vi "Sim Camera.vi"() -> ()   [LabVIEW 2012]
uses:
  Program Files (x86)/National Instruments/LabVIEW 2012/examples/robotics/Simulator/Traffic/Auto Driving/Auto Starter Kit.ctl
  <vilib>/vision/Image Controls.llb/IMAQ Image.ctl
  <vilib>/robotics/Steering/Differential Steering Frame/NI_Robotics_Differential Steering Frame.lvclass
  <instrlib>/DC Motor Controller/HAIOL/DC Motor Controller.lvclass
  <vilib>/Platform/TimedLoop/XDataNode/timing_clust.ctl
  <vilib>/Platform/TimedLoop/XDataNode/nitl_modes.ctl
  <vilib>/Platform/TimedLoop/XDataNode/wakeup.ctl
  <vilib>/robotics/Simulator/Interface/Simulator References/Get Sensor Reference.vi
  <vilib>/Platform/TimedLoop/XDataNode/XDataNode.xnode
  <vilib>/Platform/TimedLoop/XDataNode/XDNodeRunTimeDep.lvlib
  <resource>/objmgr/LVODE.rc
  <vilib>/robotics/Simulator/NI_Robotics_Simulator.lvlib
panel:
  out "VI Name":string
  out "Camera on Starter Kit 1.0":refnum<vi>(3d-picture)
  in  "error in":errorcluster
  out "error out":errorcluster
  in  "stop?":bool caption="Stop (F)"
  out "Image Out":T1(plugin-control)
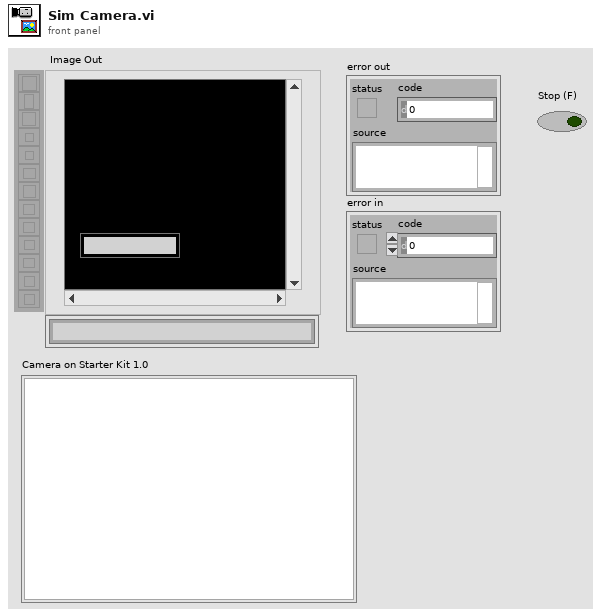
[diagram p1: front panel]
types:
  T1 = typedef "IMAQ Image.ctl" = refnum<image>
  T2 = typedef "Auto Starter Kit.ctl" = cluster{"Camera Image":T1, "Light Detect Dst":T1, "Path Detect Dst":T1, "Camera":refnum<k20>, "3D Picture":refnum<vi>, "Steering Frame":refnum<class "NI_Robotics_Differential Steering Frame.lvclass">, "Left Motor Controller":refnum<class "DC Motor Controller.lvclass">, "Right Motor Controller":refnum<class "DC Motor Controller.lvclass">}
  T3 = cluster{"Robot":string, "Sensors":string[], "Joints":string[], "Actuators":string[], "Robot Components":string[]}[]
  T4 = cluster{"Robot":string, "Sensors":string[], "Joints":string[], "Actuators":string[], "Robot Components":string[]}
  T5 = typedef "XDNodeRunTimeDep.lvlib/timing_clust.ctl" = cluster{"Expected End [f-1]":u64, "Actual End [f-1]":u64, "Finished Late? [f-1]":bool, "Expected End [i-1]":u64, "Actual End [i-1]":u64, "Finished Late? [i-1]":bool, "Expected Start [i]":u64, "Actual Start [i]":u64, "Expected Start [f]":u64, "Actual Start [f]":u64, "Source Name":string, "Structure Name":string, "Period":i64, "Deadline":i64, "Offset":i64, "Start":i64, "Priority":i32, "Timeout":i32, "Mode":T6, "Wakeup Reason":T7, "Error":errorcluster, "Source Type":string, "Secondary Source Type":string, "Global End Time":u64, "Global Start Time":u64, "Frame Duration":u64, "Iteration Duration":u64, "Assigned CPU":i32, "I/O Scan Engine Mode":u32}
  T6 = typedef "XDNodeRunTimeDep.lvlib/nitl_modes.ctl" = enum32{"No Change", "Process missed periods, maintain original phase", "Discard missed periods, maintain original phase", "Process missed periods, ignore original phase", "Discard missed periods, ignore original phase"}
  T7 = typedef "XDNodeRunTimeDep.lvlib/wakeup.ctl" = enum32{"Normal", "Aborted", "Asynchronous wakeup", "Timing source error", "Timed loop error", "Timeout"}
  T8 = cluster{"Position[0]":sgl, "Position[1]":sgl, "Position[2]":sgl}
  T9 = cluster{"Target[0]":sgl, "Target[1]":sgl, "Target[2]":sgl}
  T10 = cluster{"UpDirection[0]":sgl, "UpDirection[1]":sgl, "UpDirection[2]":sgl}
  T11 = typedef "imagedata.ctl" = cluster{"image type":i32, "image depth":i32, "image":u8[], "mask":u8[], "colors":u32[], "Rectangle":cluster{"left":i16, "top":i16, "right":i16, "bottom":i16}}
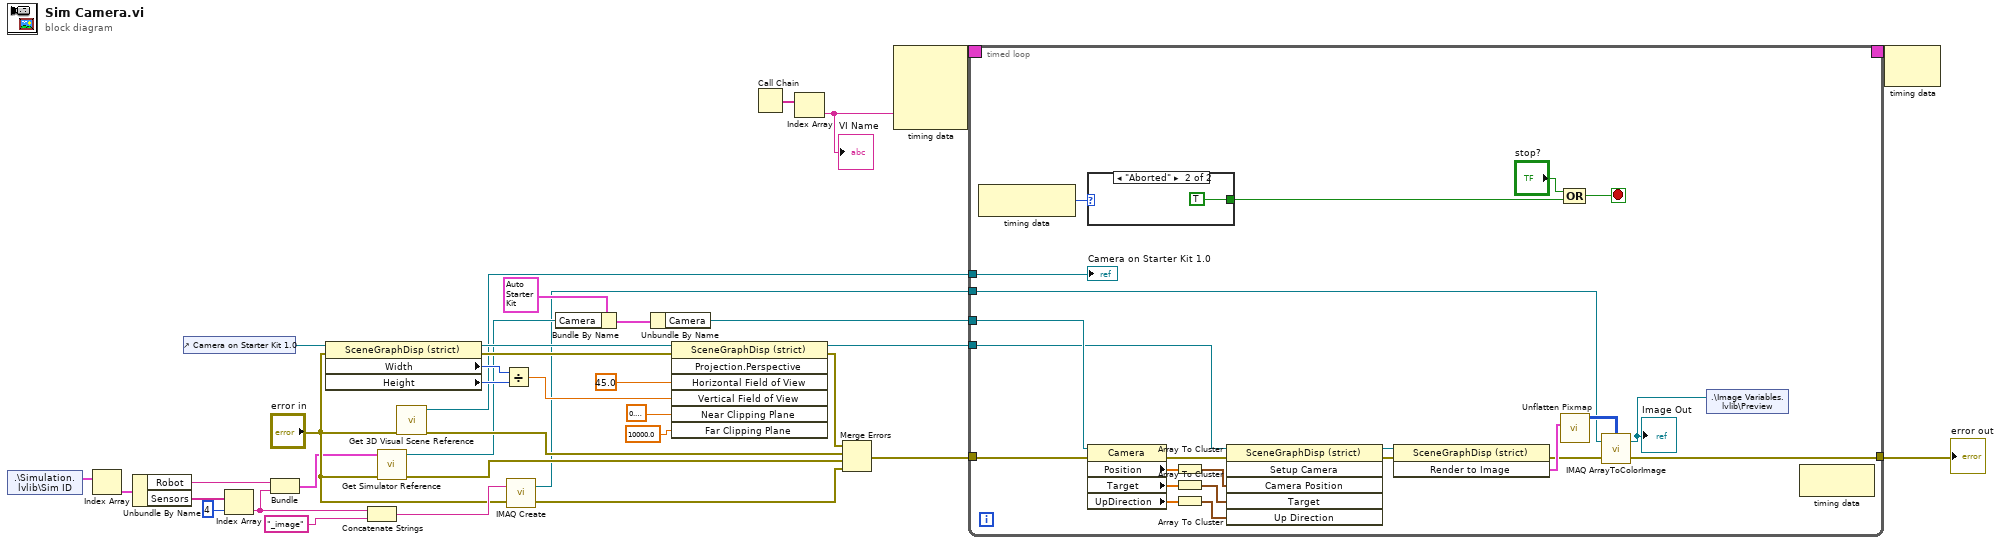
[diagram p0: block diagram]
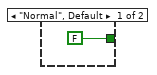
[diagram p2: hidden frame]
diagram:
  n1 = shared-variable ".\\Simulation.lvlib\\Sim ID"() -> (w9:T3)  [unwired: 1 in, 1 out]
  n2 = Index Array(array=w9) -> (element=w8:T4)  [unwired: 1 in]
  n3 = Unbundle By Name(w8) -> ("Robot"=w5:string, "Sensors"=w7:string[])
  n4 = control-ref of="Camera on Starter Kit 1.0"() -> (w25:refnum<vi>)
  n5 = Index Array(array=w7, index=4) -> (element=w4:string)
  n6 = Bundle("Robot"=w5, w4) -> (w3:cluster{"Robot":string, string})  [unwired: 1 in]
  n7 = property on="Property Node" class="SceneGraphDisp (strict)"(reference=w25, error in="error in") -> (reference out=w26:refnum<vi>, error out=w33:errorcluster, "Width"=w31:u32, "Height"=w32:u32)
  n8 = Concatenate Strings(w4, "_image" ("Image Name")) -> (w14:string)
  n9 = call-poly <vilib>:"Get Simulator Reference.vi"("error in (no error)"="error in", "device ID"=w3) -> ("error out"=w20:errorcluster, "sensor ref"=w16:refnum<k20>)  [unwired: 8 in]
  n10 = call <vilib>:"Get 3D Visual Scene Reference.vi"("error in"="error in") -> ("error out"=w22:errorcluster, "scene ref"=w24:refnum<vi>)  [unwired: 9 in]
  n11 = Divide(x=w31, y=w32) -> (x/y=w28:dbl)
  n12 = call "IMAQ Create"("Image Name"=w14, "error in (no error)"="error in") -> ("New Image"=w10:T1, "error out"=w11:errorcluster)  [unwired: 2 in, 1 out]
  n13 = Bundle By Name(cluster=T2 {"Camera Image"=refnum, "Light Detect Dst"=refnum, "Path Detect Dst"=refnum, "Camera"=refnum, "3D Picture"=refnum, "Steering Frame"=refnum, "Left Motor Controller"=refnum, "Right Motor Controller"=refnum} ("Auto Starter Kit"), "Camera"=w16) -> (w17:T2)
  n14 = Unbundle By Name(w17) -> ("Camera"=w15:refnum<k20>)
  n15 = invoke on="Invoke Node" class="SceneGraphDisp (strict)" method="Projection.Perspective"(reference=w26, error in=w33, "Horizontal Field of View"=sgl 45.0 ("Field of View"), "Vertical Field of View"=w28, "Near Clipping Plane"=sgl 0.2, "Far Clipping Plane"=sgl 10000.0) -> (reference out=w19:refnum<vi>, error out=w23:errorcluster)  [unwired: 1 in, 5 out]
  n16 = Call Chain() -> (call chain=w2:string[])
  n17 = Index Array(array=w2) -> (element=w1:string)  [unwired: 1 in]
  "VI Name" <- w1
  n18 = Merge Errors(w23, w22, w20, w11) -> (w21:errorcluster)
  n19 = node-c288(w1) -> (w36:T5)  [unwired: 3 in]
  n20 = timed-loop {
    timing: w36 -> [_]
    timing-out: [_] -> w35
    tunnel: w21 -> [w47]
    tunnel: [w46] -> w34
    tunnel: w24 -> [w45]
    tunnel: w15 -> [w44]
    tunnel: w19 -> [w43]
    tunnel: w10 -> [w41]
    stop <- w37 stop-if-true
    n21 = node-c288() -> (w40:T7)  [unwired: 1 in]
    n22 = case shown="\"Aborted\"" w40 {
      tunnel: [FALSE TRUE] -> w39
      frame "Normal", Default {
      }
      frame "Aborted" {
      }
    }
    n23 = property class="Camera"(reference=w44, error in=w47) -> (error out=w59:errorcluster, "Position"=w54:sgl[], "Target"=w52:sgl[], "UpDirection"=w50:sgl[])  [unwired: 1 out]
    n24 = Array To Cluster(array=w54) -> (cluster=w53:T8)
    n25 = Array To Cluster(array=w52) -> (cluster=w51:T9)
    n26 = Array To Cluster(array=w50) -> (cluster=w49:T10)
    n27 = invoke class="SceneGraphDisp (strict)" method="Setup Camera"(reference=w43, error in=w59, "Camera Position"=w53, "Target"=w51, "Up Direction"=w49) -> (reference out=w58:refnum<vi>, error out=w57:errorcluster)  [unwired: 1 in, 4 out]
    n28 = invoke class="SceneGraphDisp (strict)" method="Render to Image"(reference=w58, error in=w57) -> (error out=w55:errorcluster, "Get Image"=w56:T11)  [unwired: 1 in, 1 out]
    n29 = call <vilib>:"Unflatten Pixmap.vi"("image data"=w56) -> ("24-bit pixmap"=w42:u32[][])  [unwired: 4 in, 6 out]
    n30 = Compound Arithmetic op=OR("stop?", w39) -> (w37:bool)
    n31 = call "IMAQ ArrayToColorImage"("Image Pixels (U32)"=w42, "Image"=w41, "error in (no error)"=w55) -> ("Image Out"=w48:T1, "error out"=w46:errorcluster)  [unwired: 2 in]
    "Image Out" <- w48
    n32 = shared-variable ".\\Image Variables.lvlib\\Preview"(w48) -> ()  [unwired: 1 in, 1 out]
    n33 = node-c288() -> ()  [unwired: 1 in, 1 out]
    "Camera on Starter Kit 1.0" <- w45
  }
  "error out" <- w34
  n34 = node-c288(w35) -> ()  [unwired: 1 out]
